vi "PostStop - Permeability (SubVI).vi"(8 "error in (no error)":errorcluster, 11 "Cluster in in":T1 {"M Event" items=["Stop", "Running", "PID", "Up Limit", "Down Limit", "Load Limit"]; "Test Type" items=["Please Select", "Triaxial Shear", "Triaxial UU", "Shearbox", "Permeability", "Consolidation (Stepped Loading)/Swelling", "Saturation (Incremental)", "User Defined", "UCT", "Isotropic Consolidation", "Swelling Pressure"]; "Data"."Test Type" items=["Please Select", "Triaxial Shear", "Triaxial UU", "Shearbox", "Permeability", "Consolidation (Stepped Loading)/Swelling", "Saturation (Incremental)", "User Defined", "UCT", "Isotropic Consolidation", "Swelling Pressure"]}) -> (0 "error out":errorcluster, 2 "Enum":T10, 3 "Cluster out":T1 {"M Event" items=["Stop", "Running", "PID", "Up Limit", "Down Limit", "Load Limit"]; "Test Type" items=["Please Select", "Triaxial Shear", "Triaxial UU", "Shearbox", "Permeability", "Consolidation (Stepped Loading)/Swelling", "Saturation (Incremental)", "User Defined", "UCT", "Isotropic Consolidation", "Swelling Pressure"]; "Data"."Test Type" items=["Please Select", "Triaxial Shear", "Triaxial UU", "Shearbox", "Permeability", "Consolidation (Stepped Loading)/Swelling", "Saturation (Incremental)", "User Defined", "UCT", "Isotropic Consolidation", "Swelling Pressure"]})   [LabVIEW 2019]
uses:
  Controls/RunTest - State.ctl
  Controls/RunTest - Data Structure.ctl
  Controls/Test Panel - Data Structure.ctl
  Controls/Station - Test Type.ctl
  <vilib>/Utility/miscctls.llb/LVRowAndColumnTypeDef.ctl
  Controls/RunTest - Calculate Data.ctl
  <vilib>/httpClient/ClientHandle.ctl
  Controls/RunTest - Start Condition.ctl
  Controls/RunTest - Stop Condition.ctl
  Controls/UDP - Event.ctl
  <vilib>/httpClient/LabVIEWHTTPClient.lvlib
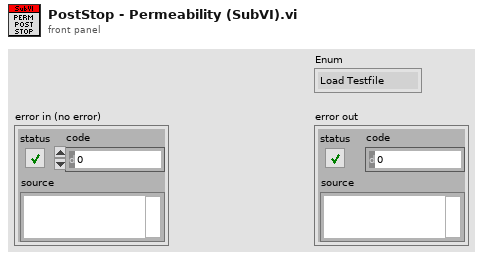
[diagram p1: front panel]
types:
  T1 = typedef "RunTest - Data Structure.ctl" = cluster{"Test Plan":string[], "PlanRow":i32, "Device Name":string[], "Timeout":i32, "Start?":bool, "Pause?":bool, "IP Address":string[], "LogRow":i32, "Logtype":u16, "Log Elapse":sgl, "Data":T2, "Stop log?":bool, "tdms":refnum<k34>, "Sensor Data":sgl[], "Start time":timestamp, "Prev Log Elapse":u32, "Plot":u16, "X-Axis":u16[], "Y-Axis":u16[], "XY":cluster{"X":dbl, "Y":dbl}[][], "End Stage?":bool, "1run":bool, "Condition":u16[], "Start Con":bool, "Log Con":bool, "Stop Con":bool, "Start Elapse":dbl, "Start Load":dbl, "Motor":i32, "StartRow":i32, "number log":i32, "Dir":bool, "Start time test":timestamp, "Auto":bool, "Check return?":bool, "Inv":cluster{"M":i32[], "Bool":bool[]}, "tdms temp":refnum<k34>, "Zero?":bool, "Plot Timer":dbl, "1st Run":bool, "TDMS Path":path, "MaxLoad":dbl, "Log Timer":sgl[], "Test Type":T3, "Log Sensor":string[], "Save?":bool, "1st Log":bool, "Y-Axis 2":u16[], "On Y-Axis 2":bool, "Decimal":u8[], "Init":cluster{"PWP TS":sgl, "Load TS":sgl, "Volume TS":sgl, "Disp TS":sgl, "CP":sgl, "Vol In":sgl, "Vol Out":sgl, "Load UCT":sgl, "Disp UCT":sgl, "PWP Sat":sgl, "CP Sat":sgl, "Volume IsoCons":sgl, "PWP IsoCons":sgl, "PWP TUU":sgl, "Load TUU":sgl, "Volume TUU":sgl, "Disp TUU":sgl, "Load Cons":sgl, "Disp Cons":sgl, "Volume Sat":sgl, "Vertical Load SB":sgl, "Vertical Disp SB":sgl, "H Disp SB":sgl, "H Load SB":sgl}, "Calc":T5, "Device Index":i32[], "Channel Index":i32[], "http ref":T6, "fileid":string, "Step Cons":cluster{"V Stress":sgl, "H Settlement":sgl}, "RunTest":bool, "Graph Last":i32, "Init?":bool, "Datalog":bool[], "Start":T7, "Stop":T8, "Running?":bool, "StartTime":dbl, "Log Prev Time":dbl, "KeyName":string[], "Test RunTime":dbl, "Log Prev Axial":dbl, "M Event":T9[], "Last Log":bool, "popup":bool, "PreStart UU":bool, "PreStart Sat":bool}
  T2 = typedef "Test Panel - Data Structure.ctl" = cluster{"Station":string, "Sample ID":string, "Job No":string, "Job Description":string, "Filename":string, "Test Type":T3, "Speciment No":string, "Depth":string, "Height":string, "Diameter/Length":string, "Weight":string, "Test Parameter":string, "Station[]":string[], "Edit Pos":T4, "Edit Pos Prev":T4, "Area":string, "Path":string}
  T3 = typedef "Station - Test Type.ctl" = u16
  T4 = typedef "LVRowAndColumnTypeDef.ctl" = cluster{"Row":i32, "Column":i32}
  T5 = typedef "RunTest - Calculate Data.ctl" = cluster{"TS":cluster{"Change PWP":sgl, "Change Vol":sgl, "Axial Load":sgl, "CiL":sgl, "Deviator":sgl, "Axial Strain":sgl, "MaxDeviator":sgl}, "TUU":cluster{"Change PWP":sgl, "Axial Load":sgl, "CiL":sgl, "Deviator":sgl, "Axial Strain":sgl, "MaxDeviator":sgl}, "Sat":cluster{"B Value":sgl, "PWP Diss":sgl, "CPP":sgl, "CV":sgl}, "Per":cluster{"Change Vol In":sgl, "Change Vol Out":sgl, "Mean Vol":sgl, "Gradient Pressure":sgl, "Outlet Flow":sgl, "Inlet Flow":sgl, "I X1":sgl, "I X2":sgl, "I Y1":sgl, "I Y2":sgl, "O X1":sgl, "O X2":sgl, "O Y1":sgl, "O Y2":sgl}, "Step Cons":cluster{"V Stress":sgl, "H Settlement":sgl, "Total H Settle":sgl, "Prev Total H":sgl}, "UCT":cluster{"ALC":sgl, "H Change":sgl, "Deviator":sgl, "Axial Strain":sgl, "V Stress":sgl, "MaxDeviator":sgl}, "ISO Cons":cluster{"CPP":sgl, "PWP Diss":sgl, "CV":sgl}, "SB":cluster{"Speci LenC":sgl, "Shear Strain":sgl, "H LC":sgl, "Normal Stress":sgl, "Shear Stress":sgl, "MaxShear":sgl}}
  T6 = typedef "LabVIEWHTTPClient.lvlib/ClientHandle.ctl" = refnum<k1>
  T7 = typedef "RunTest - Start Condition.ctl" = cluster{"Cons":cluster{"VS":dbl, "Delay":bool, "No Delay":dbl}, "Sat":cluster{"CP":dbl, "BP":dbl, "StartBP":bool, "Target CP":bool, "Target BP":bool}, "Iso":cluster{"BP":dbl}, "TS":cluster{"SS":dbl, "Engage":bool, "ES":dbl, "LC":dbl, "PreStart":bool, "Trig SS":bool, "Drain":dbl}, "TUU":cluster{"SS":dbl, "Engage":bool, "ES":dbl, "LC":dbl, "PreStart":bool, "Trig SS":bool, "CP":dbl, "Delay Value":dbl, "Delay":bool, "CP PID":bool}, "UCT":cluster{"SS":dbl, "Engage":bool, "ES":dbl, "LC":dbl, "PreStart":bool, "Trig SS":bool}, "Enable?":bool, "SB":cluster{"SS":dbl, "Engage":bool, "ES":dbl, "LC":dbl, "PreStart":bool, "Trig SS":bool, "VS":dbl, "Delay Value":dbl, "Delay":bool, "VS PID":bool}, "Perm":cluster{"DP":dbl}}
  T8 = typedef "RunTest - Stop Condition.ctl" = cluster{"Cons":cluster{"Select":i32, "Disp":dbl, "Time":dbl, "Time2":dbl, "Disp 2":dbl, "Time Cond":dbl, "Last Disp":dbl, "Swell":bool}, "Sat":cluster{"Select":i32, "PP":dbl, "Time":dbl, "VC":dbl, "Time2":dbl, "Time Cond":dbl, "Last PP":dbl, ".B":bool, "B":dbl, "Last Vc":dbl, "Time Cond 2":dbl, "Time3":dbl, "Time Cond 3":dbl}, "Iso":cluster{"PP":dbl, "Time":dbl, "VC":dbl, "Time2":dbl, "Time Cond":dbl, "Last Vc":dbl, ".PP":bool, "Time Cond 2":dbl, "Select":i32}, "TS":cluster{"Axial":dbl, ".MaxDev":bool, "MaxDev Value":dbl, "Return":bool, "Reset":bool, "Prev Time":dbl, "PostStop Run":bool, "CP Stop":bool, "BP Stop":bool, "PostStop Trig":bool, "Reset Value":dbl, "BPTrig":bool, "CPTrig":bool, "VLCTrig":bool}, "TUU":cluster{"Axial":dbl, ".MaxDev":bool, "MaxDev Value":dbl, "Return":bool, "Reset":bool, "Prev Time":dbl, "PostStop Run":bool, "CP Stop":bool, "BP Stop":bool, "PostStop Trig":bool, "Reset Value":dbl, "BPTrig":bool, "CPTrig":bool, "VLCTrig":bool}, "UCT":cluster{"Axial":dbl, ".MaxDev":bool, "MaxDev Value":dbl, "Return":bool, "Reset":bool, "Prev Time":dbl, "PostStop Run":bool, "CP Stop":bool, "BP Stop":bool, "PostStop Trig":bool}, "Enable?":bool, "SB":cluster{"Shear":dbl, ".MaxShear":bool, "MaxShear Value":dbl, "Return":bool, "Reset":bool, "Prev Time":dbl, "PostStop Run":bool, "CP Stop":bool, "BP Stop":bool, "PostStop Trig":bool, "Reset Value":dbl, "BPTrig":bool, "CPTrig":bool, "VLCTrig":bool}, "Perm":cluster{"Max Time":bool, "Reset":bool, "PostStop Run":bool, "Ratio":bool, "Reset Value":dbl, "Time":dbl, "RatioTime":dbl, "RatioMore":dbl, "RatioLess":dbl, "Time Cond":dbl, "Time Cond 2":dbl, "Prev IF":dbl, "Prev OF":dbl, "PostStop Trig":bool, "BP Trig":bool, "DP Stop":bool, "BP Stop":bool, "CP Stop":bool, "CP Trig":bool}, "SP":cluster{".Max Time":bool, ".Time":bool, "Time":dbl, "MaxTime":dbl, "Time Cond":dbl, "Max Time Cond":dbl, "Stress":dbl}}
  T9 = typedef "UDP - Event.ctl" = u16
  T10 = typedef "RunTest - State.ctl" = enum16{"Load Testfile", "Notifier", "Init", "Idle", "Load", "Read DB", "Run", "Pause", "Stop", "Check Start", "Check Stop", "Check Post Stop", "Check Log", "EndStage", "Data View", "Display", "Graph", "Graph Old", "Close", "Stop PID", "Check Limit", "Auto", "Up", "Log", "Zero", "Machine Control", "Save Report"}
  T11 = enum32{"Please Select", "Triaxial Shear", "Triaxial UU", "Shearbox", "Permeability", "Consolidation", "Saturation", "User Defined", "UCT", "Iso Consolidation"}
  T12 = cluster{"Target Load":sgl, "Target Disp":sgl, "Rate":sgl, "Speed":sgl}
  T13 = enum16{"None", "Run Target", "Run Ramp", "Run Disp"}
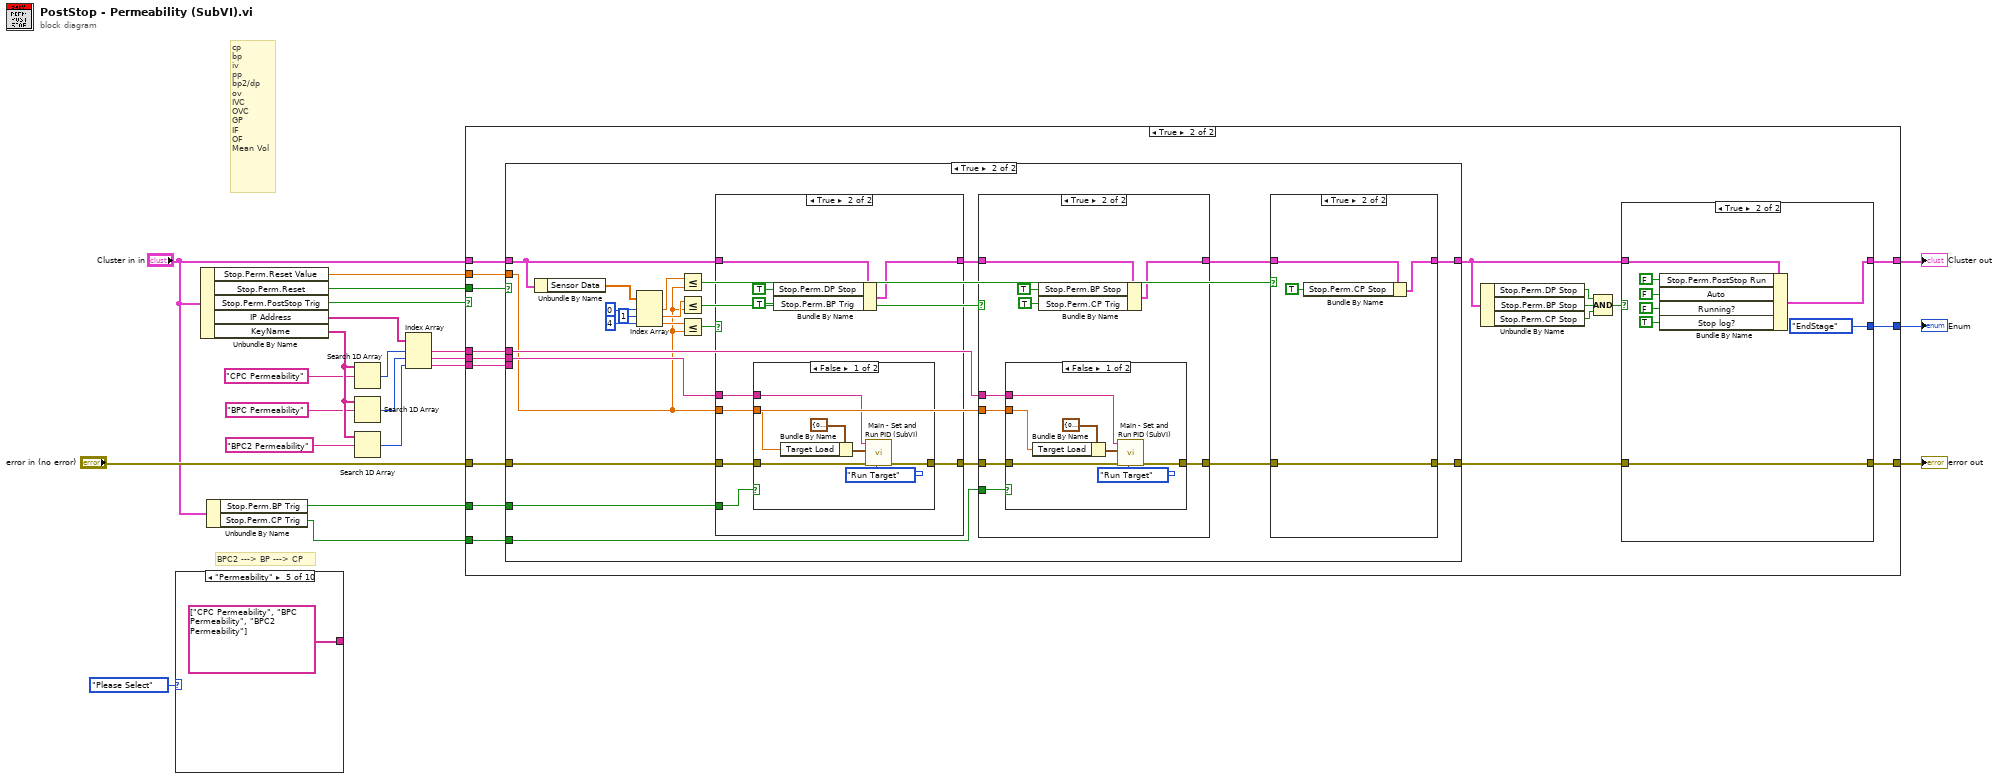
[diagram p0: block diagram]
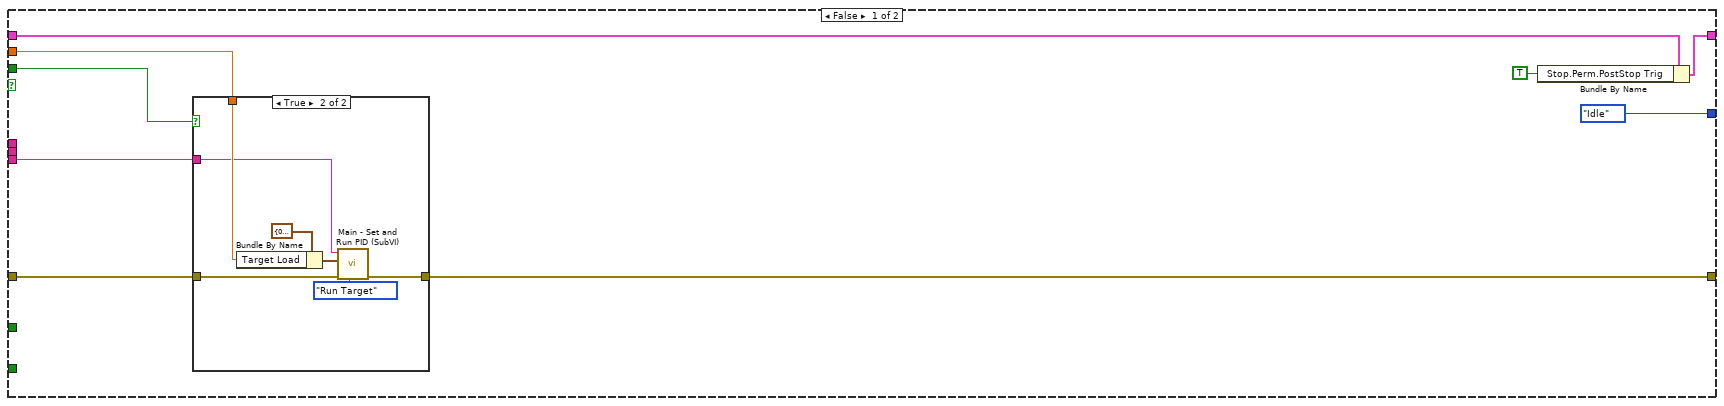
[diagram p2: hidden frame]
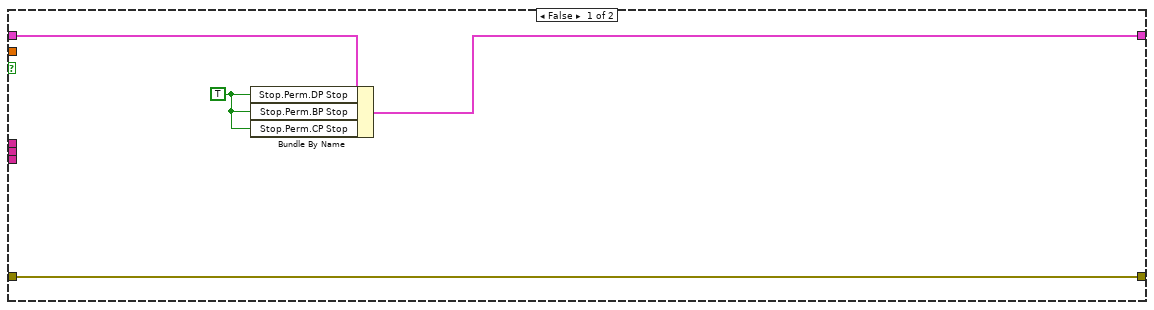
[diagram p4: hidden frame]
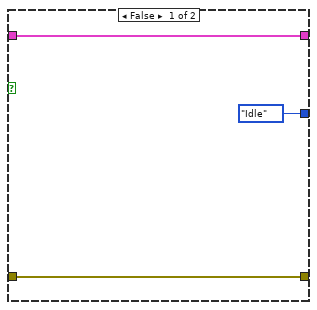
[diagram p10: hidden frame]
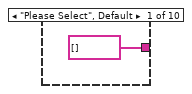
[diagram p11: hidden frame]
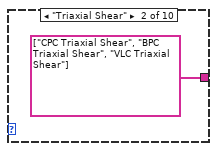
[diagram p12: hidden frame]
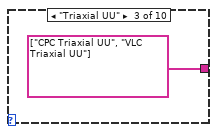
[diagram p13: hidden frame]
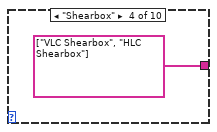
[diagram p14: hidden frame]
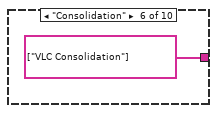
[diagram p15: hidden frame]
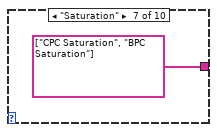
[diagram p16: hidden frame]
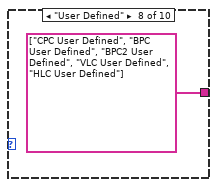
[diagram p17: hidden frame]
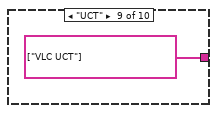
[diagram p18: hidden frame]
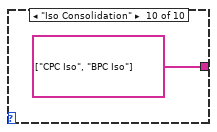
[diagram p19: hidden frame]
diagram:
  # "cp\nbp\niv\npp\nbp2/dp\nov\nIVC\nOVC\nGP\nIF\nOF\nMean Vol"
  # "BPC2 ---> BP ---> CP"
  n1 = case shown="\"Permeability\"" T11."Please Select" ("Sub Tab") {
    tunnel: [string[] [] string[] ["CPC Triaxial Shear", "BPC Triaxial Shear", "VLC Triaxial Shear"] string[] ["CPC Triaxial UU", "VLC Triaxial UU"] string[] ["VLC Shearbox", "HLC Shearbox"] string[] ["CPC Permeability", "BPC Permeability", "BPC2 Permeability"] string[] ["VLC Consolidation"] string[] ["CPC Saturation", "BPC Saturation"] string[] ["CPC User Defined", "BPC User Defined", "BPC2 User Defined", "VLC User Defined", "HLC User Defined"] string[] ["VLC UCT"] string[] ["CPC Iso", "BPC Iso"]] -> _
    frame "Please Select", Default {
    }
    frame "Triaxial Shear" {
    }
    frame "Triaxial UU" {
    }
    frame "Shearbox" {
    }
    frame "Permeability" {
    }
    frame "Consolidation" {
    }
    frame "Saturation" {
    }
    frame "User Defined" {
    }
    frame "UCT" {
    }
    frame "Iso Consolidation" {
    }
  }
  n2 = Unbundle By Name("Cluster in in") -> ("Stop.Perm.Reset Value"=w13:dbl, "Stop.Perm.Reset"=w12:bool, "Stop.Perm.PostStop Trig"=w11:bool, "IP Address"=w22:string[], "KeyName"=w21:string[])
  n3 = Unbundle By Name("Cluster in in") -> ("Stop.Perm.BP Trig"=w5:bool, "Stop.Perm.CP Trig"=w1:bool)
  n4 = Search 1D Array(1D array=w21, element="CPC Permeability" ("String")) -> (index of element=w17:i32)  [unwired: 1 in]
  n5 = Search 1D Array(1D array=w21, element="BPC Permeability" ("String")) -> (index of element=w18:i32)  [unwired: 1 in]
  n6 = Search 1D Array(1D array=w21, element="BPC2 Permeability" ("String")) -> (index of element=w20:i32)  [unwired: 1 in]
  n7 = Index Array(array=w22, index #1=w17, index #2=w18, index #3=w20) -> (element #1=w9:string, element #2=w8:string, element #3=w7:string)
  n8 = case shown="True" w11 {
    tunnel: [w39 w62] -> w4
    tunnel: "Cluster in in" -> [w41 w63]
    tunnel: [w35 w60] -> w2
    tunnel: "error in (no error)" -> [w34 w67]
    tunnel: w9 -> [_ w66]
    tunnel: w8 -> [_ w65]
    tunnel: [RunTest_-_State."Idle" w64] -> w3
    tunnel: w7 -> [w33 w56]
    tunnel: w12 -> [w37 w55]
    tunnel: w13 -> [w36 w58]
    tunnel: w5 -> [_ w57]
    tunnel: w1 -> [_ w54]
    frame False {
      n9 = case shown="True" w37 {
        tunnel: w34 -> [w42 w46]
        tunnel: [w42 w44] -> w35
        tunnel: w36 -> [_ w45]
        tunnel: w33 -> [_ w43]
        frame False {
        }
        frame True {
          n10 = Bundle By Name(cluster=T12 {"Target Load"=0.0, "Target Disp"=0.0, "Rate"=0.0, "Speed"=0.0} ("Test"), "Target Load"=w45) -> (w47:T12)
          n11 = call "Main - Set and Run PID (SubVI).vi"("Action"=T13."Run Target", "error in (no error)"=w46, "Test"=w47, "IP Address"=w43) -> ("error out"=w44:errorcluster)  [unwired: 7 in]
        }
      }
      n12 = Bundle By Name(cluster=w41, "Stop.Perm.PostStop Trig"=TRUE ("Stop.TS.PostStop Run")) -> (w39:T1)
    }
    frame True {
      n13 = case shown="True" w55 {
        tunnel: w67 -> [w69 w94]
        tunnel: w66 -> [_ w78]
        tunnel: w65 -> [_ w83]
        tunnel: w63 -> [w71 w93]
        tunnel: [w70 w81] -> w61
        tunnel: [w69 w79] -> w59
        tunnel: w58 -> [_ w73]
        tunnel: w57 -> [_ w84]
        tunnel: w56 -> [_ _]
        tunnel: w54 -> [_ w77]
        frame False {
          w68 = TRUE ("Stop.Perm.DP Stop")
          n14 = Bundle By Name(cluster=w71, "Stop.Perm.DP Stop"=w68, "Stop.Perm.BP Stop"=w68, "Stop.Perm.CP Stop"=w68) -> (w70:T1)
        }
        frame True {
          n15 = Unbundle By Name(w93) -> ("Sensor Data"=w92:sgl[])
          n16 = Index Array(array=w92, index #1=0 ("index"), index #2=1 ("index"), index #3=4 ("index")) -> (element #1=w74:sgl, element #2=w85:sgl, element #3=w86:sgl)
          n17 = Less Or Equal?(x=w74, y=w73) -> (x <= y?=w72:bool)
          n18 = Less Or Equal?(x=w85, y=w73) -> (x <= y?=w75:bool)
          n19 = Less Or Equal?(x=w86, y=w73) -> (x <= y?=w87:bool)
          n20 = case shown="True" w87 {
            tunnel: w94 -> [w121 w123]
            tunnel: [w121 w128] -> w89
            tunnel: w93 -> [w120 w130]
            tunnel: [w120 w129] -> w88
            tunnel: w83 -> [_ w127]
            tunnel: w73 -> [_ w126]
            tunnel: w84 -> [_ w124]
            frame False {
            }
            frame True {
              n21 = case shown="False" w124 {
                tunnel: w123 -> [w134 w138]
                tunnel: [w133 w138] -> w128
                tunnel: w127 -> [w132 _]
                tunnel: w126 -> [w131 _]
                frame False {
                  n22 = Bundle By Name(cluster=T12 {"Target Load"=0.0, "Target Disp"=0.0, "Rate"=0.0, "Speed"=0.0} ("Test"), "Target Load"=w131) -> (w137:T12)
                  n23 = call "Main - Set and Run PID (SubVI).vi"("Action"=T13."Run Target", "error in (no error)"=w134, "Test"=w137, "IP Address"=w132) -> ("error out"=w133:errorcluster)  [unwired: 7 in]
                }
                frame True {
                }
              }
              n24 = Bundle By Name(cluster=w130, "Stop.Perm.DP Stop"=TRUE, "Stop.Perm.BP Trig"=TRUE ("Stop.TS.CPTrig")) -> (w129:T1)
            }
          }
          n25 = case shown="True" w75 {
            tunnel: w89 -> [w102 w108]
            tunnel: [w102 w107] -> w80
            tunnel: w88 -> [w101 w110]
            tunnel: [w101 w109] -> w82
            tunnel: w78 -> [_ w106]
            tunnel: w73 -> [_ w105]
            tunnel: w77 -> [_ w104]
            frame False {
            }
            frame True {
              n26 = case shown="False" w104 {
                tunnel: w108 -> [w115 w119]
                tunnel: [w114 w119] -> w107
                tunnel: w106 -> [w113 _]
                tunnel: w105 -> [w112 _]
                frame False {
                  n27 = Bundle By Name(cluster=T12 {"Target Load"=0.0, "Target Disp"=0.0, "Rate"=0.0, "Speed"=0.0} ("Test"), "Target Load"=w112) -> (w118:T12)
                  n28 = call "Main - Set and Run PID (SubVI).vi"("Action"=T13."Run Target", "error in (no error)"=w115, "Test"=w118, "IP Address"=w113) -> ("error out"=w114:errorcluster)  [unwired: 7 in]
                }
                frame True {
                }
              }
              n29 = Bundle By Name(cluster=w110, "Stop.Perm.BP Stop"=TRUE ("Stop.TS.BP Stop"), "Stop.Perm.CP Trig"=TRUE) -> (w109:T1)
            }
          }
          n30 = case shown="True" w72 {
            tunnel: w80 -> [w96 w97]
            tunnel: [w96 w97] -> w79
            tunnel: w82 -> [w95 w99]
            tunnel: [w95 w98] -> w81
            frame False {
            }
            frame True {
              n31 = Bundle By Name(cluster=w99, "Stop.Perm.CP Stop"=TRUE ("Stop.TS.BP Stop")) -> (w98:T1)
            }
          }
        }
      }
      n32 = Unbundle By Name(w61) -> ("Stop.Perm.DP Stop"=w53:bool, "Stop.Perm.BP Stop"=w52:bool, "Stop.Perm.CP Stop"=w51:bool)
      n33 = Compound Arithmetic op=AND(w53, w52, w51) -> (w50:bool)
      n34 = case shown="True" w50 {
        tunnel: [RunTest_-_State."Idle" RunTest_-_State."EndStage"] -> w64
        tunnel: [w140 w146] -> w62
        tunnel: w61 -> [w140 w148]
        tunnel: [w139 w142] -> w60
        tunnel: w59 -> [w139 w142]
        frame False {
        }
        frame True {
          n35 = Bundle By Name(cluster=w148, "Stop.Perm.PostStop Run"=FALSE ("Stop.TS.PostStop Run"), "Auto"=FALSE, "Running?"=FALSE, "Stop log?"=TRUE) -> (w146:T1)
        }
      }
    }
  }
  "Enum" <- w3
  "error out" <- w2
  "Cluster out" <- w4
